vi "Analyse error.vi"(8 "error in (no error)":errorcluster, 11 "IErrorHandler in":refnum<class "AbortHandler MsgPack.lvclass">) -> (0 "error out":errorcluster, 3 "IErrorHandler out":refnum<class "AbortHandler MsgPack.lvclass">)   [LabVIEW 2020, in "wamplv.lvlib" / "AbortHandler MsgPack.lvclass"]
uses:
  AbortHandler MsgPack.lvclass
  AbortHandler MsgPack.lvclass/AbortHandler MsgPack.ctl
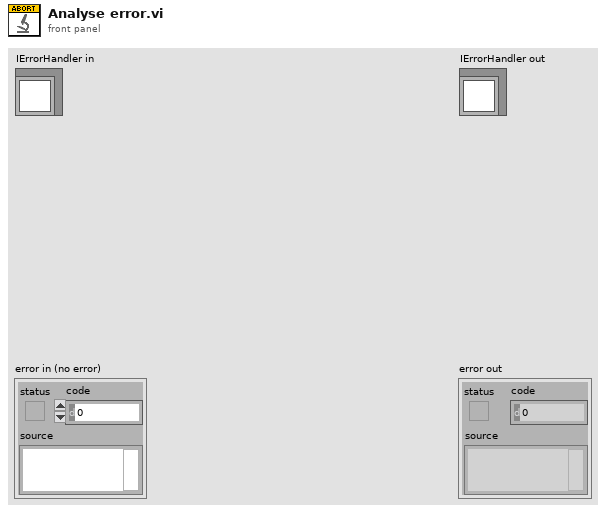
[diagram p1: front panel]
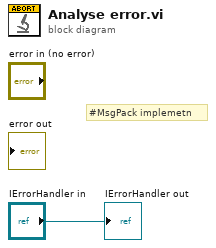
[diagram p0: block diagram]
diagram:
  # "#MsgPack implemetn"
  "IErrorHandler out" <- "IErrorHandler in"
